vi "FTW-CodeGen-Prototype.vi"(0 "REPLACED_Data":variant, 11 "REPLACED_error in":errorcluster) -> (4 "REPLACED_JSON String":string, 15 "REPLACED_error out":errorcluster)   [LabVIEW 2012]
uses:
  src/Container/FTW-Container.lvclass
panel:
  # "Inputs"
  # "Outputs"
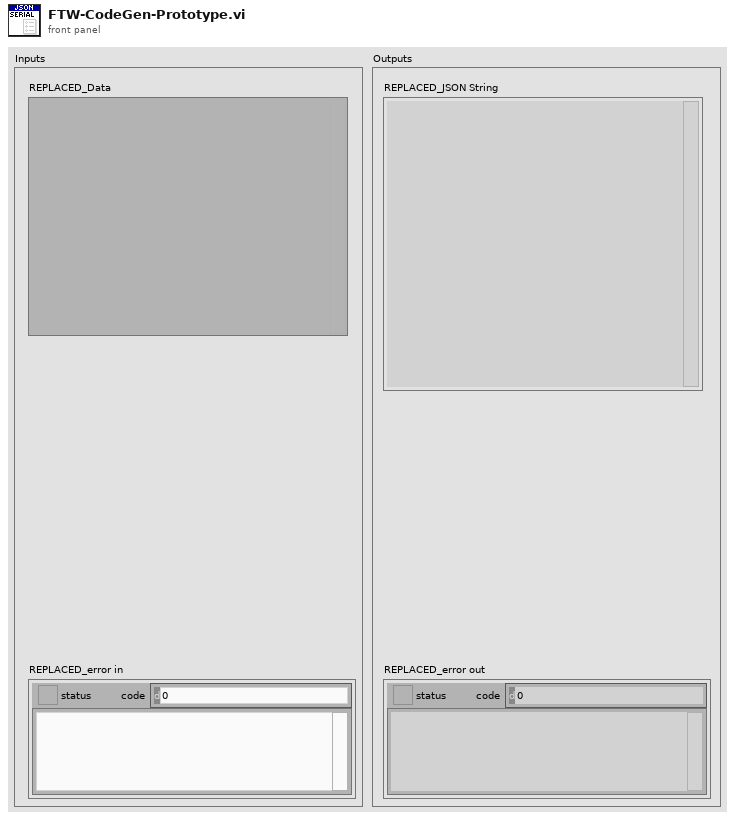
[diagram p1: front panel]
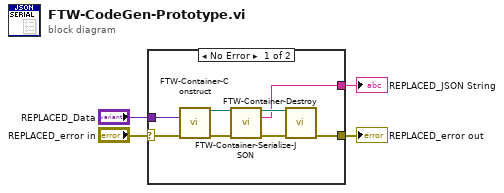
[diagram p0: block diagram]
diagram:
  n1 = case shown="No Error" "REPLACED_error in" {
    selector: "REPLACED_error in" -> [w7 w13]
    tunnel: "REPLACED_Data" -> [w12 _]
    tunnel: [w6 w13] -> w3
    tunnel: [w5 _] -> w1
    frame No Error {
      n2 = call "FTW-Container-Construct.vi"("LabVIEW Data Structure"=w12, "error in"=w7) -> ("Container"=w11:refnum<class "FTW-Container.lvclass">, "error out"=w9:errorcluster)  [unwired: 12 in]
      n3 = call "FTW-Container-Serialize-JSON.vi"("Container"=w11, "error in"=w9) -> ("Container out"=w10:refnum<class "FTW-Container.lvclass">, "Serialized Container"=w5:string, "error out"=w8:errorcluster)  [unwired: 11 in]
      n4 = call "FTW-Container-Destroy.vi"("Container"=w10, "error in"=w8) -> ("error out"=w6:errorcluster)  [unwired: 13 in]
    }
    frame Error {
    }
  }
  "REPLACED_error out" <- w3
  "REPLACED_JSON String" <- w1
